vi "DAQ Initialization 4 MM.vi"(8 "error in":errorcluster, 11 "classes in":T2) -> (0 "error out":errorcluster, 3 "classes out":T2)   [LabVIEW 2011]
uses:
  Controls/Class Objects.ctl
  Modules/File/Configuration/Configuration.lvclass
  Modules/Hardware/Power Supply/Power Supply.lvclass
  Modules/Hardware/Mass Flow Controller/Mass Flow Controller.lvclass
  Modules/Hardware/Valve Controller/Valve Controller.lvclass
  Modules/Hardware/Vapour Generator/Vapour Generator.lvclass
  Modules/Hardware/PID/PID.lvclass
  Modules/Hardware/Multimeter/Multimeter.lvclass
  Modules/File/TDMS/TDMS.lvclass
  Controls/DAQ Type.ctl
  Controls/Display Mode.ctl
  Controls/User Interface Action.ctl
  Functional Global Data/Globals.ctl
  Functional Global Data/Run Data.ctl
  Modules/File/TDMS/File Level.ctl
  Controls/TDMS File Handling.ctl
  Functional Global Data/Device Params Global.ctl
panel:
  in  "Experiment Type":T1
  in  "property names":string[](array[string])=["Notes", "Experiment Type", "Power Line Cycles"]
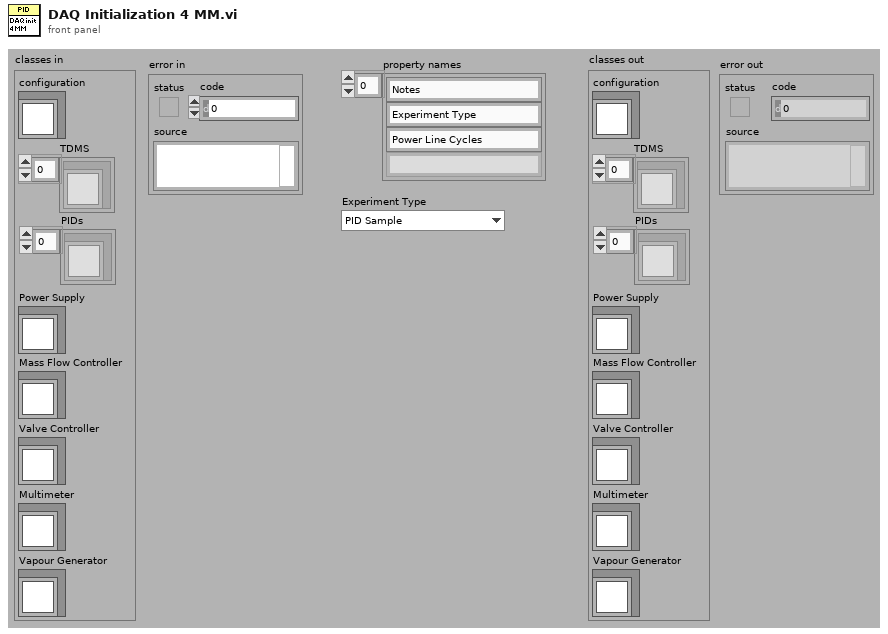
[diagram p1: front panel]
types:
  T1 = typedef "DAQ Type.ctl" = enum16{"PID Sample", "PID with PS Challenge", "PID with MFC Challenge", "Multimeter Sample", "Multimeter with MFC Challenge"}
  T2 = typedef "Class Objects.ctl" = cluster{"configuration":refnum<class "Configuration.lvclass">, "TDMS":refnum<class "TDMS.lvclass">[], "Power Supply":refnum<class "Power Supply.lvclass">, "Mass Flow Controller":refnum<class "Mass Flow Controller.lvclass">, "Valve Controller":refnum<class "Valve Controller.lvclass">, "Multimeter":refnum<class "Multimeter.lvclass">, "Vapour Generator":refnum<class "Vapour Generator.lvclass">, "PIDs":refnum<class "PID.lvclass">[]}
  T3 = typedef "Display Mode.ctl" = enum16{"Sample", "Run"}
  T4 = typedef "User Interface Action.ctl" = enum16{"Initialize", "Data Acquisition Disable", "Data View Disable", "Sample Set", "Sample Set 2D Data", "Sample Set x0 & dx", "Sample Add", "Sample Set Cursor", "Sample Set Offset & Multiplier", "Sample Set Axis Labels", "Sample Parameters Disabled", "Sample Parameters Update", "Run Update", "Run Set Offset & Multiplier", "Run Set Axis Labels", "Run Set Cursor", "Run Set Disabled", "Run Parameters Update", "Run Parameters Disabled", "Run Number Set", "Run Number Set Range", "Run Number Set Disabled", "Sample Number Set", "Sample Number Set Range", "Notes Set Value", "Update Plot", "Set Plot Parameters", "Update Concentration Plot", "Time Set", "Clear DAQ Display", "Clear Analysis Display", "Status Bar Set", "Progress Bar Set", "Display Mode Set", "Experiment Type Set", "Analysis Plot Average Set", "Stop"}
  T5 = typedef "Globals.ctl" = enum16{"Initialize", "Get DAQ Params", "Get Data Display Params", "Set DAQ Params", "Set Data Display Params"}
  T6 = typedef "Run Data.ctl" = enum16{"Initialize", "Add Sample Channel", "Set Run", "Get Number of Runs", "Set Run Params", "Get Spectrum", "Get Run Params", "Get Sample Params", "Get History", "Get Averaged History", "Get Run Param Names", "Set Run Param Names", "Get Sample Param Names", "Set Sample Param Names", "Get MFC Flow Rate Challenge Profile", "Get History Average"}
  T7 = typedef "TDMS.lvclass/File Level.ctl" = enum16{"File", "Group", "Channel"}
  T8 = typedef "TDMS File Handling.ctl" = enum16{"Add TDMS File", "Get Active TDMS File", "Set Active TDMS File", "Set Active TDMS File Index"}
  T9 = typedef "Device Params Global.ctl" = enum16{"Initialize", "Get Device Settings", "Get Device Connections", "Set Device Settings", "Set Device Connections", "Get All Device Properties"}
  T10 = enum8{"Enabled", "Disabled", "Disabled and Grayed Out"}
  T11 = typedef "Data Acquisition Parameters.ctl" = cluster{"Experiment Type":T1, "Experiment Name":string, "Operator Name":string, "Notes":string, "TDMS File Path":path, "Data Acquisition State":bool, "PID Voltage Sweep":T12, "MFC Challenge Profile - Heaviside Step":T13, "MFC Challenge Profile":T14, "MFC Challenge Profile - Staircase":T15}
  T12 = typedef "PID Voltage Seep Settings.ctl" = cluster{"Voltage Step (V)":dbl, "Voltage Range (V)":cluster{u16, u16}, "Time Step (s)":dbl, "Voltage Step Direction":enum16{"High 2 Low", "Low 2 High"}}
  T13 = typedef "MFC Challenge Profile - Heaviside Step.ctl" = cluster{"Valve Open Duration":u16, "MFC Flow Rate":dbl, "Valve Open Repeats":u16, "Valve Open Start":u16}
  T14 = typedef "MFC Challen Profile Type.ctl" = enum16{"Heaviside", "Staircase"}
  T15 = typedef "MFC Challenge Profile - Staircase.ctl" = cluster{"Step Time Duration":u16, "Step Flow Rate":dbl, "Steps":u16, "Valve Open Start":u16, "Recovery":bool, "Repeats":u16}
  T16 = typedef "Device Settings.ctl" = cluster{"PID":cluster{"B-M PID":T17, "INL PID":T18}, "Power Supply":cluster{"Source Value":dbl, "Source Value Units":T19, "Source Mode":T20, "Limits":T21, "Output":bool}, "Mass Flow Controller":cluster{"MFC Flow Rate":dbl, "MFC Valve Status":T24}, "Valve Controller":cluster{"Valve Assembly":T25}, "Multimeter":cluster{"Agilent 3458A":cluster{"Measurement Configuration":T27, "Measurement Integration":T28}}, "Vapour Generator":cluster{"Owlstone Permeation Tube":T29, "Owlstone GEN-SYS Setpoints":T31}}
  T17 = typedef "Baseline Mocon piD-Tech plus.lvclass/Settings.ctl" = cluster{"Detector Sampling Frequency":dbl}
  T18 = typedef "INL PID.lvclass/Settings.ctl" = cluster{"Sampling Frequency":dbl, "Integration Time":dbl, "Integration Periods":u8, "Grid Voltage":dbl}
  T19 = typedef "Power Supply.lvclass/Source Units.ctl" = enum16{"volts", "millivolts", "microvolts", "amps", "milliamps", "microamps", "nanoamps"}
  T20 = typedef "Power Supply.lvclass/Source Mode.ctl" = enum16{"Volts", "Current"}
  T21 = typedef "Power Supply.lvclass/Protection Limits.ctl" = cluster{"Voltage Limit":dbl, "Voltage Limit Units":T22, "Current Limit":dbl, "Current Limit Units":T23, "Voltage Trip/Cmpl":dbl, "Voltage Trip/Cmpl Units":T22, "Current Trip/Cmpl":dbl, "Current Trip/Cmpl Units":T23}
  T22 = typedef "Power Supply.lvclass/Voltage Units.ctl" = enum16{"volts", "millivolts", "microvolts"}
  T23 = typedef "Power Supply.lvclass/Current Units.ctl" = enum16{"amps", "milliamps", "microamps", "nanoamps"}
  T24 = typedef "Mass Flow Controller.lvclass/Valve Status.ctl" = enum16{"Open", "Closed"}
  T25 = typedef "Valve Controller.lvclass/Valve Assembly.ctl" = cluster{"Valve 1":T26, "Valve 2":T26, "Valve 3":T26, "Valve 4":T26, "Valve 5":T26}
  T26 = typedef "Valve Controller.lvclass/Status.ctl" = u16
  T27 = typedef "Agilent 3458A.lvclass/Measurement Configuration.ctl" = cluster{"Function":enum16{"DC Voltage", "AC Voltage", "AC + DC Voltage", "DC Current", "AC Current", "AC + DC Current", "2-Wire Resistance", "4-Wire Resistance", "Frequency", "Period", "Direct Sampling DC", "Direct Sampling AC", "Sub-Sampling DC", "Sub-Sampling AC"}, " Manual Resolution":enum16{"4.5", "5.5", "6.5", "7.5", "8.5"}, "Frequency Source":enum16{"AC + DC Current", "AC + DC Voltage", "AC Current", "AC Voltage"}, "Auto Range":enum16{"OFF", "ON", "ONCE"}}
  T28 = typedef "Agilent 3458A.lvclass/Measurement Integration.ctl" = cluster{"Power Line Cycles":dbl}
  T29 = typedef "Owlstone GEN-SYS.lvclass/Permeation Tube.ctl" = cluster{"Tube":T30, "Molecular Weight":dbl, "Calibration Temperature\n(Celcius)":i32, "Permeation Rate \n(ng/min)":i32}
  T30 = typedef "Owlstone GEN-SYS.lvclass/Permeation Tube Gas.ctl" = enum16{"Isobutylene 27 Nov 2012", "Ammonia 29 Sep 2012", "DMMP Tube A 3 July 2014", "DMMP Tube B 3 July 2014"}
  T31 = typedef "Owlstone GEN-SYS.lvclass/Gen-Sys Setpoints.ctl" = cluster{"OVG-4":cluster{"Oven Temperature":i32, "Sample Flow Rate":i32, "Split Flow Status":u16, "Split Flow Rate":i32}, "OHG-4":cluster{"Wet Air Flow":i32}}
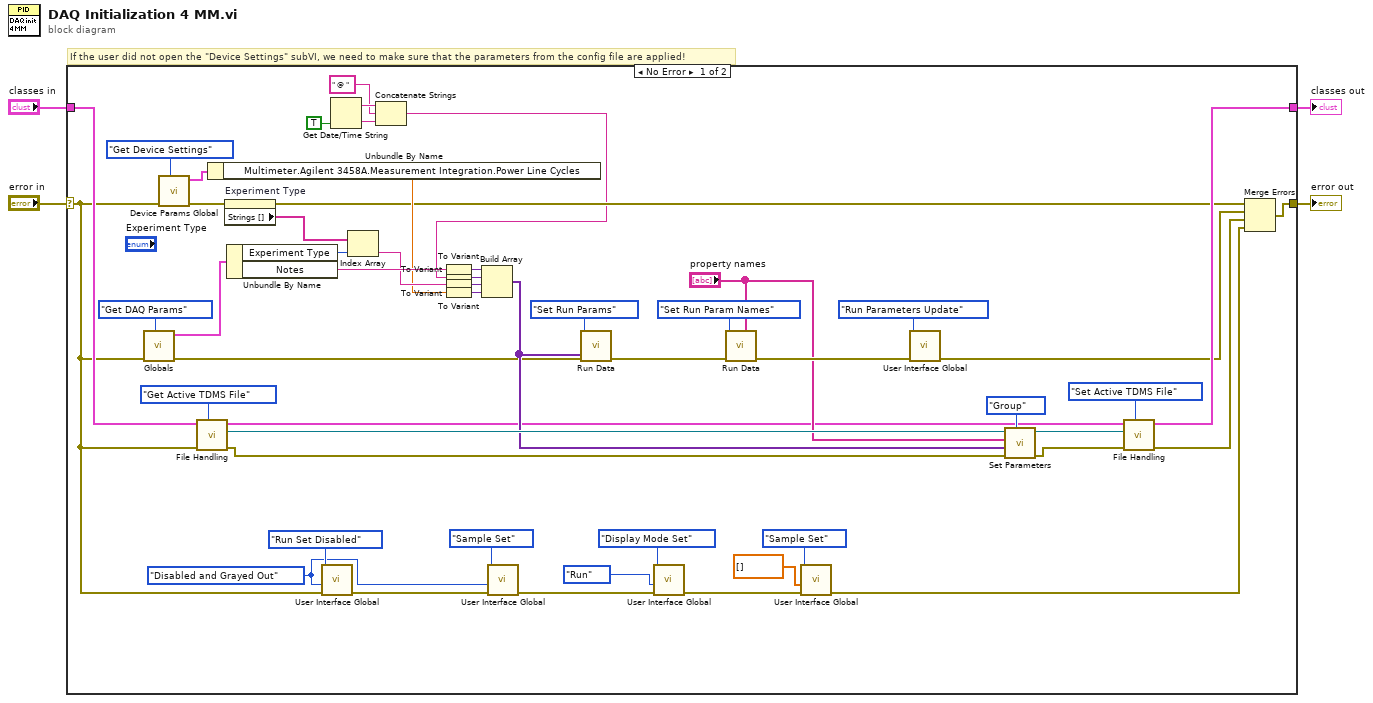
[diagram p0: block diagram]
diagram:
  # "If the user did not open the \"Device Settings\" subVI, we need to make sure that the parameters from the config file are applied!"
  n1 = case shown="No Error" "error in" {
    selector: "error in" -> [w31 w59]
    tunnel: [w49 w59] -> w4
    tunnel: "classes in" -> [w54 w58]
    tunnel: [w48 w58] -> w1
    frame No Error {
      w8 = T10."Disabled and Grayed Out" ("Disabled")
      n2 = call "Globals.vi"("action"=Globals."Get DAQ Params", "error in"=w31) -> ("error out"=w6:errorcluster, "Data Acquisition"=w41:T11)  [unwired: 7 in, 1 out]
      n3 = call "Device Params Global.vi"("action"=Device_Params_Global."Get Device Settings", "error in"=w31) -> ("error out"=w19:errorcluster, "Device Settings OUT"=w56:T16)  [unwired: 7 in, 1 out]
      n4 = call "File Handling.vi"("TDMS File Handling"=TDMS_File_Handling."Get Active TDMS File", "error in"=w31, "Class objects"=w54) -> ("error out"=w36:errorcluster, "TDMS File"=w51:refnum<class "TDMS.lvclass">, "Class objects"=w24:T2)  [unwired: 6 in]
      n5 = Unbundle By Name(w56) -> ("Multimeter.Agilent 3458A.Measurement Integration.Power Line Cycles"=w25:dbl)
      n6 = property on="Experiment Type" class="Enum (strict)"(error in=w19) -> (error out=w18:errorcluster, "Strings []"=w29:string[])  [unwired: 1 in, 1 out]
      n7 = Unbundle By Name(w41) -> ("Experiment Type"=w28:T1, "Notes"=w39:string)
      n8 = call "User Interface Global.vi"("error in"=w31, "data1"=w8, "action"=User_Interface_Action."Run Set Disabled" ("Action")) -> ("error out"=w22:errorcluster)  [unwired: 8 in]
      n9 = Get Date/Time String(want seconds? (F)=TRUE) -> (date string=w15:string, time string=w14:string)  [unwired: 2 in]
      n10 = Index Array(array=w29, index=w28) -> (element=w27:string)
      n11 = Concatenate Strings(w15, " @ " ("string"), w14) -> (w12:string)
      n12 = To Variant(anything=w39) -> (Variant=w42:variant)
      n13 = To Variant(anything=w12) -> (Variant=w17:variant)
      n14 = To Variant(anything=w27) -> (Variant=w30:variant)
      n15 = To Variant(anything=w25) -> (Variant=w26:variant)
      n16 = Build Array(w42, w17, w30, w26) -> (w37:variant[])
      n17 = call "User Interface Global.vi"("error in"=w22, "data1"=w8, "action"=User_Interface_Action."Sample Set" ("Action")) -> ("error out"=w10:errorcluster)  [unwired: 8 in]
      n18 = call "Run Data.vi"("Params 1D IN"=w37, "error in"=w6, "action"=Run_Data."Set Run Params" ("Action")) -> ("error out"=w45:errorcluster)  [unwired: 5 in, 3 out]
      n19 = call "User Interface Global.vi"("error in"=w10, "data1"=Display_Mode."Run" ("Display Mode"), "action"=User_Interface_Action."Display Mode Set" ("Action")) -> ("error out"=w7:errorcluster)  [unwired: 8 in]
      n20 = call "Run Data.vi"("Param Names IN"="property names", "error in"=w45, "action"=Run_Data."Set Run Param Names" ("Action")) -> ("error out"=w43:errorcluster)  [unwired: 5 in, 3 out]
      n21 = call "User Interface Global.vi"("error in"=w7, "data1"=dbl[] [], "action"=User_Interface_Action."Sample Set" ("Action")) -> ("error out"=w5:errorcluster)  [unwired: 8 in]
      n22 = call "User Interface Global.vi"("error in"=w43, "action"=User_Interface_Action."Run Parameters Update" ("Action")) -> ("error out"=w34:errorcluster)  [unwired: 9 in]
      n23 = call-dynamic "Set Parameters.vi"("File Level"=File_Level."Group", "error in (no error)"=w36, "property values"=w37, "property names"="property names", "TDMS.lvclass in"=w51) -> ("error out"=w35:errorcluster, "TDMS.lvclass out"=w50:refnum<class "TDMS.lvclass">)  [unwired: 5 in]
      n24 = call "File Handling.vi"("TDMS File Handling"=TDMS_File_Handling."Set Active TDMS File", "error in"=w35, "TDMS File"=w50, "Class objects"=w24) -> ("error out"=w33:errorcluster, "Class objects"=w48:T2)  [unwired: 5 in, 1 out]
      n25 = Merge Errors(w18, w34, w33, w5) -> (w49:errorcluster)
    }
    frame Error {
    }
  }
  "error out" <- w4
  "classes out" <- w1
